vi "hasPacketIdentifier.vi"(11 "SUBSCRIBE in":refnum<class "SUBSCRIBE.lvclass">) -> (2 "As Packet Identifier":bool, 3 "SUBSCRIBE out":refnum<class "SUBSCRIBE.lvclass">)   [LabVIEW 2013, in "SUBSCRIBE.lvclass"]
uses:
  SUBSCRIBE.lvclass
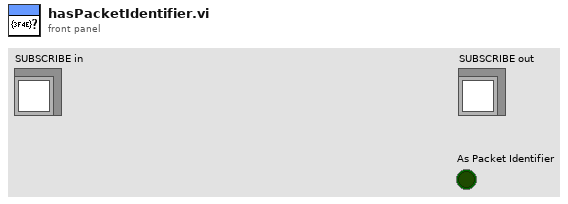
[diagram p1: front panel]
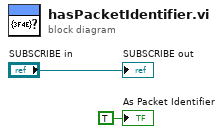
[diagram p0: block diagram]
diagram:
  "SUBSCRIBE out" <- "SUBSCRIBE in"
  "As Packet Identifier" <- TRUE ("As Packet Identifier")
